vi "INST_PS_MEAS_1.0.0.vi"(4 "Use OPC?(T)":bool=TRUE, 6 "Instrument Select (Output 1)":string(combo)="OUT1", 8 "error in (no error)":errorcluster, 9 "Measurement Type (Voltage)":string(combo)="MEAS:VOLT?", 11 "VISA session":refnum<visa-resource-name>) -> (0 "error out":errorcluster, 2 "Measurement":dbl format="%.2p", 3 "dup VISA session":refnum<visa-resource-name>)   [LabVIEW 2018]
doc: "This VI takes a measurement on the output signal and returns the measured value."
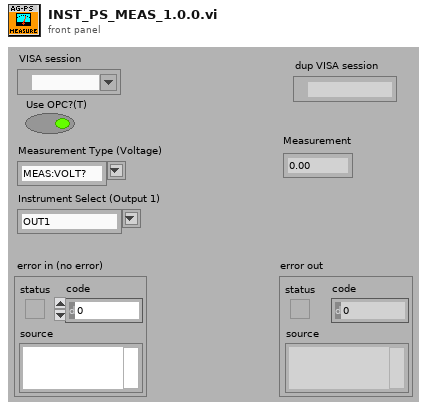
[diagram p1: front panel]
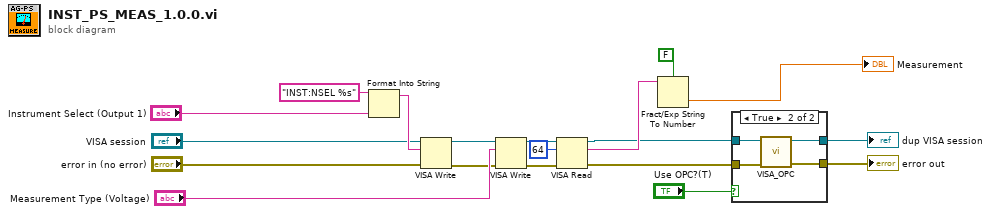
[diagram p0: block diagram]
diagram:
  n1 = Format Into String(format string="INST:NSEL %s", "Instrument Select (Output 1)") -> (resulting string=w10:string)  [unwired: 2 in, 1 out]
  n2 = VISA Write(VISA resource name="VISA session", write buffer=w10, error in (no error)="error in (no error)") -> (VISA resource name out=w7:refnum<visa-resource-name>, error out=w8:errorcluster)  [unwired: 1 out]
  n3 = VISA Write(VISA resource name=w7, write buffer="Measurement Type (Voltage)", error in (no error)=w8) -> (VISA resource name out=w15:refnum<visa-resource-name>, error out=w19:errorcluster)  [unwired: 1 out]
  n4 = VISA Read(VISA resource name=w15, byte count=u32 64, error in (no error)=w19) -> (VISA resource name out=w2:refnum<visa-resource-name>, read buffer=w17:string, error out=w5:errorcluster)  [unwired: 1 out]
  n5 = Fract/Exp String To Number(use system decimal point (T)=FALSE, string=w17) -> (number=→"Measurement":dbl)  [unwired: 2 in, 1 out]
  n6 = case shown="True" "Use OPC?(T)" {
    tunnel: w5 -> [w20 w25]
    tunnel: [w20 w24] -> w4
    tunnel: [w21 w23] -> w3
    tunnel: w2 -> [w21 w22]
    frame False {
    }
    frame True {
      n7 = call "VISA_OPC.vi"("error in"=w25, "Session In"=w22) -> ("error out"=w24:errorcluster, "Session Out"=w23:refnum<visa-resource-name>)  [unwired: 7 in, 1 out]
    }
  }
  "error out" <- w4
  "dup VISA session" <- w3
